vi "FRCts20_EspEngine_Reports_AdvancedComponents.vi"(8 "error in (no error)":errorcluster, 10 "Advanced Components":T1, 11 "httpRequestID":u32) -> (0 "error out":errorcluster, 3 "httpRequestID out":u32)   [LabVIEW 2014, in "FRCts20_EspEngine.lvlib"]
uses:
  FRCts20_EspEngine.lvlib
  TypeDefs/FRCts20_EspEngine_AdvancedComponents_Bar.ctl
  <vilib>/wsapi/subVIs/Set Integer ESP Variable.vi
  <vilib>/wsapi/NI_WebServices.lvlib
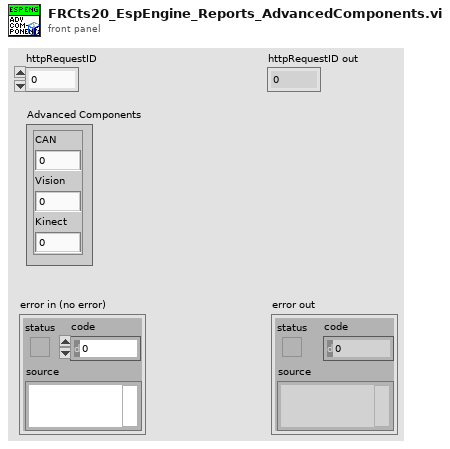
[diagram p1: front panel]
types:
  T1 = typedef "FRCts20_EspEngine.lvlib/FRCts20_EspEngine_AdvancedComponents_Bar.ctl" = cluster{"CAN":i32, "Vision":i32, "Kinect":i32}
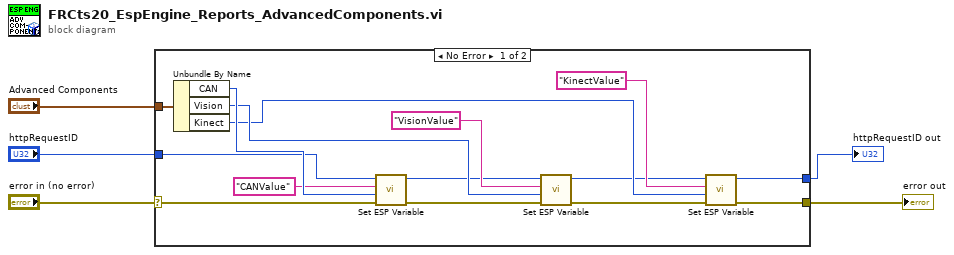
[diagram p0: block diagram]
diagram:
  n1 = case shown="No Error" "error in (no error)" {
    selector: "error in (no error)" -> [w18 w21]
    tunnel: [w9 w21] -> w5
    tunnel: "Advanced Components" -> [w20 _]
    tunnel: "httpRequestID" -> [w10 _]
    tunnel: [w8 _] -> w1
    frame No Error {
      n2 = Unbundle By Name(w20) -> ("CAN"=w19:i32, "Vision"=w15:i32, "Kinect"=w14:i32)
      n3 = call-poly <vilib>:"Set ESP Variable.vi"("error in (no error)"=w18, "value"=w19, "key"="CANValue", "httpRequestID"=w10) -> ("error out"=w17:errorcluster, "httpRequestID out"=w6:u32)  [unwired: 6 in]
      n4 = call-poly <vilib>:"Set ESP Variable.vi"("error in (no error)"=w17, "value"=w15, "key"="VisionValue", "httpRequestID"=w6) -> ("error out"=w16:errorcluster, "httpRequestID out"=w7:u32)  [unwired: 6 in]
      n5 = call-poly <vilib>:"Set ESP Variable.vi"("error in (no error)"=w16, "value"=w14, "key"="KinectValue", "httpRequestID"=w7) -> ("error out"=w9:errorcluster, "httpRequestID out"=w8:u32)  [unwired: 6 in]
    }
    frame Error {
    }
  }
  "error out" <- w5
  "httpRequestID out" <- w1
